vi "URAPILogin.vi"(2 "error in":errorcluster, 3 "Task":enum16{"Init", "Close"}(ring), 4 "Bot Settings in":T1) -> (0 "error out":errorcluster, 1 "Bot Settings out":T1)   [LabVIEW 2012]
uses:
  <userlib>/BotSpeak/VIs/Direct/BotSpeak_Control.ctl
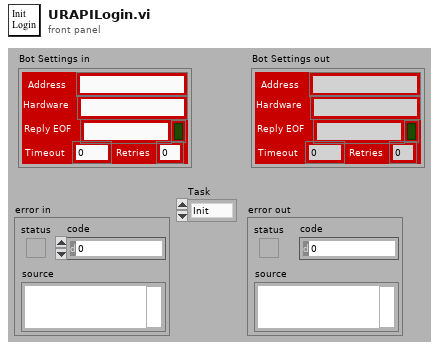
[diagram p1: front panel]
types:
  T1 = typedef "BotSpeak_Control.ctl" = cluster{"Address":string, "Reply EOF":string, "Hardware":string, "Retries":i8, "Timeout":i32, "Open?":bool}
  T2 = typedef "BotSpeak.HardwareSpecs.ctl" = cluster{"Hardware Name":string, "Hardware URL":string, "ComType":enum16{"Undefined", "Serial", "TCPIP", "Console", "EV3"}, "TCP Port":i32, "DefaultAddress":string, "Retries":i32, "Translate":enum16{"None", "Tiny", "URAPI"}, "MaxScriptSize":i32, "MaxVarNumber":i32, "StartupWait":i32, "Patience":i32, "Startup Patience":i32, "Hardware Help":string, "Com Protocol":string, "Translator":cluster{"BotSpeak CMD":string, "CMD out":string}[], "Init Code":string, "Variable Format":enum16{"INT", "FLOAT", "FIXED"}, "username":string, "password":string}
  T3 = typedef "CommState.ctl" = cluster{"Bot Settings":T4, "Initialized":bool, "Talking":bool}
  T4 = typedef "BotSpeak_Control.ctl" = cluster{"Address":string, "Reply EOF":string, "Hardware":string, "Retries":i8, "Timeout":i32}
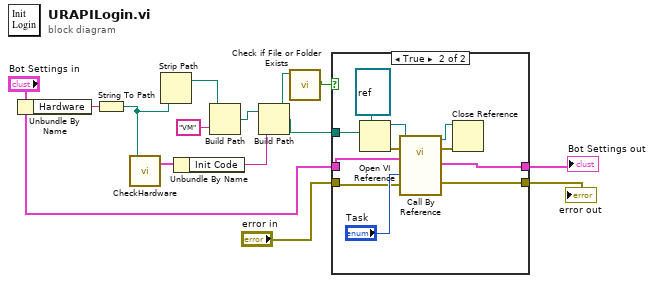
[diagram p0: block diagram]
diagram:
  n1 = Unbundle By Name("Bot Settings in") -> ("Hardware"=w3:string)
  n2 = String To Path(string=w3) -> (path=w1:path)
  n3 = call <userlib>:"CheckHardware.vi"("Hardware"=w1) -> ("HardwareSpecs"=w13:T2)  [unwired: 2 in]
  n4 = Strip Path(path=w1) -> (stripped path=w2:path)  [unwired: 1 out]
  n5 = Unbundle By Name(w13) -> ("Init Code"=w10:string)
  n6 = Build Path(base path=w2, name or relative path="VM") -> (appended path=w11:path)
  n7 = Build Path(base path=w11, name or relative path=w10) -> (appended path=w5:path)
  n8 = call <vilib>:"Check if File or Folder Exists.vi"("path"=w5) -> ("file or folder exists?"=w4:bool)  [unwired: 8 in, 2 out]
  n9 = case shown="True" w4 {
    tunnel: "Bot Settings in" -> [w15 w17]
    tunnel: "error in" -> [w14 w19]
    tunnel: [w15 w16] -> w7
    tunnel: [w14 w18] -> w6
    tunnel: w5 -> [_ w21]
    frame False {
    }
    frame True {
      n10 = Open VI Reference(type specifier VI Refnum (for type only)=refnum<vi> refnum, vi path=w21) -> (vi reference=w26:refnum<vi>, error out=w25:errorcluster)  [unwired: 4 in]
      n11 = call-by-ref "?"(reference=w26, error in=w25, "error in"=w19, "Task"="Task", "Connection in"=w17) -> (reference out=w23:refnum<vi>, error out=w24:errorcluster, 0:"error out"=w18:errorcluster, "Connection Out"=w16:T3)  [unwired: 1 out]
      n12 = Close Reference(reference=w23, error in (no error)=w24) -> ()  [unwired: 1 out]
    }
  }
  "error out" <- w6
  "Bot Settings out" <- w7
